vi "setDAQmxTaskRef.vi"(8 "error in (no error)":errorcluster, 10 "DAQmx Task Ref":refnum<k21>, 11 "niDAQmxDO.lvclass in":refnum<class "niDAQmxDO.lvclass">) -> (0 "error out":errorcluster, 3 "niDAQmxDO.lvclass out":refnum<class "niDAQmxDO.lvclass">)   [LabVIEW 2009, in "Hardware.lvlib" / "Channels.lvlib" / "niDAQmxDO.lvclass"]
uses:
  niDAQmxDO.lvclass
  niDAQmxDO.lvclass/niDAQmxDO.ctl
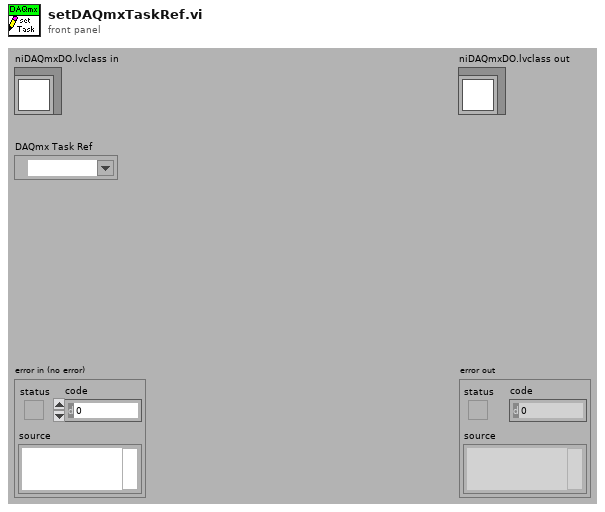
[diagram p1: front panel]
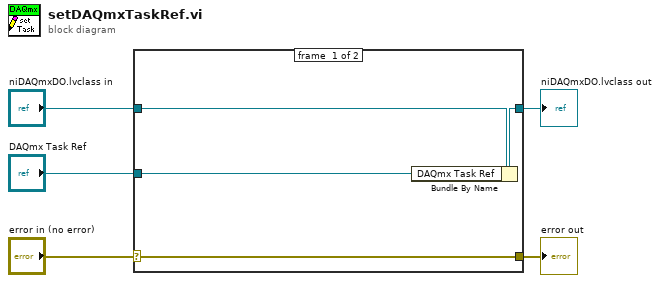
[diagram p0: block diagram]
diagram:
  n1 = case shown="No Error" "error in (no error)" {
    selector: "error in (no error)" -> [w9 w10]
    tunnel: [w9 w10] -> w4
    tunnel: [w7 w11] -> w2
    tunnel: "niDAQmxDO.lvclass in" -> [w8 w11]
    tunnel: "DAQmx Task Ref" -> [w6 _]
    frame #0 {
      n2 = Bundle By Name(cluster=w8, "DAQmx Task Ref"=w6) -> (w7:refnum<class "niDAQmxDO.lvclass">)
    }
    frame #1 {
    }
  }
  "error out" <- w4
  "niDAQmxDO.lvclass out" <- w2
